vi "Get Global Color Table.vi"(8 "error in (no error)":errorcluster caption="错误输入（无错误）", 11 "Gif Image 输入":refnum<class "Gif Image.lvclass"> caption="DNL_LabVIEW Object in") -> (0 "error out":errorcluster caption="错误输出", 3 "Gif Image 输出":refnum<class "Gif Image.lvclass"> caption="DNL_LabVIEW Object out")   [LabVIEW 2012, in "Picture Box Tools.lvlib" / "Gif Image.lvclass"]
uses:
  Gif Image.lvclass
  Gif Image.lvclass/Gif Image.ctl
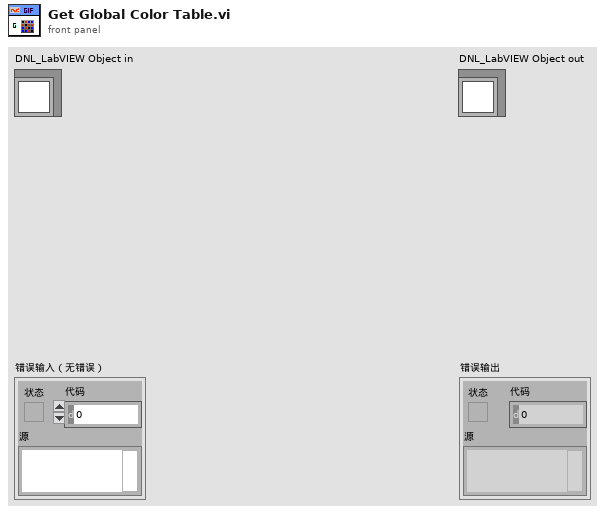
[diagram p1: front panel]
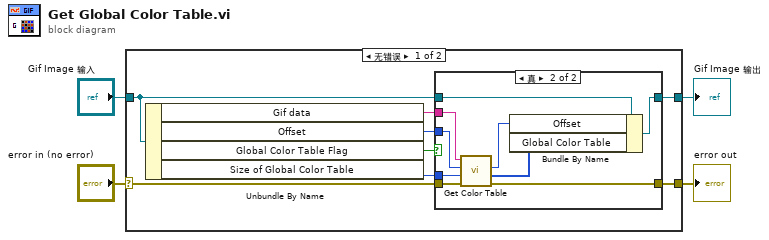
[diagram p0: block diagram]
diagram:
  n1 = case shown="无错误" "error in (no error)" {
    selector: "error in (no error)" -> [w6 w25]
    tunnel: [w5 w25] -> w3
    tunnel: [w8 w24] -> w1
    tunnel: "Gif Image 输入" -> [w9 w24]
    frame No Error {
      n2 = Unbundle By Name(w9) -> ("Gif data"=w7:string, "Offset"=w10:i32, "Global Color Table Flag"=w12:bool, "Size of Global Color Table"=w11:u8)
      n3 = case shown="真" w12 {
        tunnel: w11 -> [_ w23]
        tunnel: w10 -> [_ w21]
        tunnel: w9 -> [w14 w19]
        tunnel: [w14 w20] -> w8
        tunnel: w7 -> [_ w22]
        tunnel: w6 -> [w13 w18]
        tunnel: [w13 w17] -> w5
        frame False {
        }
        frame True {
          n4 = call "Get Color Table.vi"("错误输入"=w18, "Size of Color Table"=w23, "Offset In"=w21, "Gif data In"=w22) -> ("错误输出"=w17:errorcluster, "Color Table"=w15:u32[], "Offset Out"=w16:i32)  [unwired: 4 in, 1 out]
          n5 = Bundle By Name(cluster=w19, "Offset"=w16, "Global Color Table"=w15) -> (w20:refnum<class "Gif Image.lvclass">)
        }
      }
    }
    frame Error {
    }
  }
  "error out" <- w3
  "Gif Image 输出" <- w1
